vi "MissingInProjectCLI.vi"   [LabVIEW 2020]
uses:
  <vilib>/Wiresmith Technology/G CLI/CLI Class/CLI.lvclass
  Missing in Project Tests.lvlib
types:
  T1 = enum16{"open", "replace", "create", "open or create", "replace or create", "replace or create with confirmation"}
  T2 = enum32{"Invalid", "Standard", "Closed", "Hidden", "Minimized", "Maximized"}
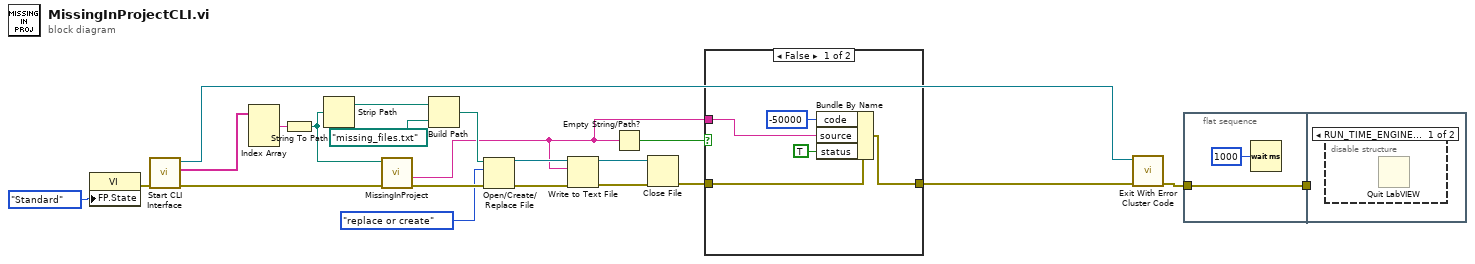
[diagram p0: block diagram]
diagram:
  n1 = property class="VI"("FP.State"=T2."Standard" ("Front Panel Window:State")) -> (error out=w21:errorcluster)  [unwired: 2 in, 1 out]
  n2 = call <vilib>:"Start CLI Interface.vi"("error in (no error)"=w21) -> ("error out"=w15:errorcluster, "Custom Parameters"=w19:string[], "CLI out"=w20:refnum<class "CLI.lvclass">)  [unwired: 7 in, 1 out]
  n3 = Index Array(array=w19) -> (element #1=w16:string)  [unwired: 3 in, 2 out]
  n4 = String To Path(string=w16) -> (path=w9:path)
  n5 = Strip Path(path=w9) -> (stripped path=w8:path)  [unwired: 1 out]
  n6 = call "MissingInProject.vi"("error in"=w15, "File Path"=w9) -> ("error out"=w10:errorcluster, "Missing Files"=w2:string)  [unwired: 7 in, 1 out]
  n7 = Build Path(base path=w8, name or relative path=path "missing_files.txt") -> (appended path=w6:path)
  n8 = Open/Create/Replace File(file path (use dialog)=w6, error in=w10, operation (0:open)=T1."replace or create") -> (refnum out=w13:refnum<file>, error out=w14:errorcluster)  [unwired: 3 in, 1 out]
  n9 = Write to Text File(file (use dialog)=w13, text=w2, error in=w14) -> (refnum out=w11:refnum<file>, error out=w12:errorcluster)  [unwired: 1 in, 1 out]
  n10 = Empty String/Path?(string/path=w2) -> (empty?=w4:bool)
  n11 = Close File(refnum=w11, error in=w12) -> (error out=w3:errorcluster)  [unwired: 1 out]
  n12 = case shown="False" w4 {
    tunnel: w3 -> [w27 w28]
    tunnel: w2 -> [w24 _]
    tunnel: [w26 w28] -> w1
    frame False {
      n13 = Bundle By Name(cluster=w27, "code"=-50000, "source"=w24, "status"=TRUE) -> (w26:errorcluster)
    }
    frame True {
    }
  }
  n14 = call <vilib>:"Exit With Error Cluster Code.vi"("error in (no error)"=w1, "CLI in"=w20) -> ("error out"=w17:errorcluster)  [unwired: 9 in]
  n15 = flat-sequence {
    tunnel: w17 -> [w30]
    tunnel: [w30] -> w18
    tunnel: w18 -> [_]
    frame #0 {
      n16 = Wait (ms)(milliseconds to wait=u32 1000) -> ()  [unwired: 1 out]
    }
    frame #1 {
      n17 = disable-structure shown="RUN_TIME_ENGINE==True" {
        frame condition #0 {
          n18 = Quit LabVIEW() -> ()  [unwired: 1 in]
        }
        frame condition #1 (active) {
        }
      }
    }
  }
